vi "ExecuteTactic.vi"(0 "object in":refnum<class "InterceptBallTactic.lvclass">, 2 "Robot in":refnum<class "Robot.lvclass">, 4 "GameRef":refnum<data-value>, 5 "error in (no error)":errorcluster) -> (14 "object out":refnum<class "InterceptBallTactic.lvclass">, 16 "Robot out":refnum<class "Robot.lvclass">, 19 "error out":errorcluster)   [LabVIEW 2023, in "InterceptBallTactic.lvclass"]
uses:
  InterceptBallTactic.lvclass
  NewSTP/NewTactics/Tactic_v2_class/Tactic_v2.lvclass
  Game_class/Game.lvclass
  Robot_class/Robot.lvclass
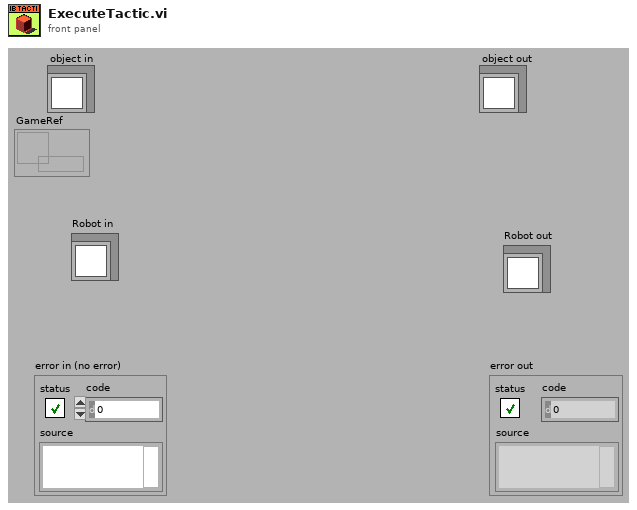
[diagram p1: front panel]
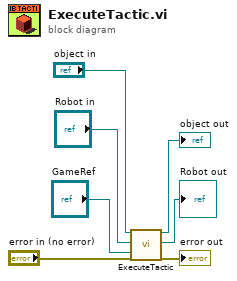
[diagram p0: block diagram]
diagram:
  n1 = call-parent "ExecuteTactic.vi"("object in"="object in", "Robot in"="Robot in", "GameRef"="GameRef", "error in (no error)"="error in (no error)") -> ("object out"=→"object out":refnum<class "InterceptBallTactic.lvclass">, "Robot out"=→"Robot out":refnum<class "Robot.lvclass">, "error out"=→"error out":errorcluster)  [unwired: 13 in]
